vi "readInXml.vi"(8 "error in (no error)":errorcluster, 10 "NativeXML out":refnum<class "NativeXML.lvclass">, 11 "deviceDataBase in":refnum<class "deviceDataBase.lvclass">) -> (0 "error out":errorcluster, 3 "deviceDataBase out":refnum<class "deviceDataBase.lvclass">)   [LabVIEW 2009, in "Tools.lvlib" / "DatabaseHelpers.lvlib" / "deviceDataBase.lvclass"]
uses:
  deviceDataBase.lvclass
  NativeXML/NativeXML.lvclass
  deviceDataBase.lvclass/deviceDataBase.ctl
  Database Objects/DeviceArray/DeviceArray.lvclass
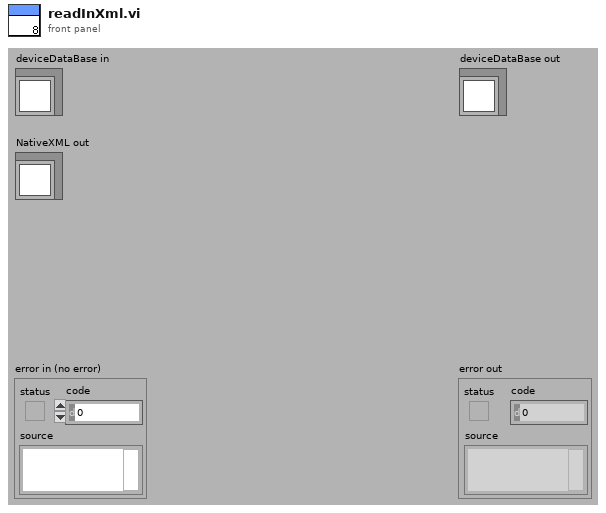
[diagram p1: front panel]
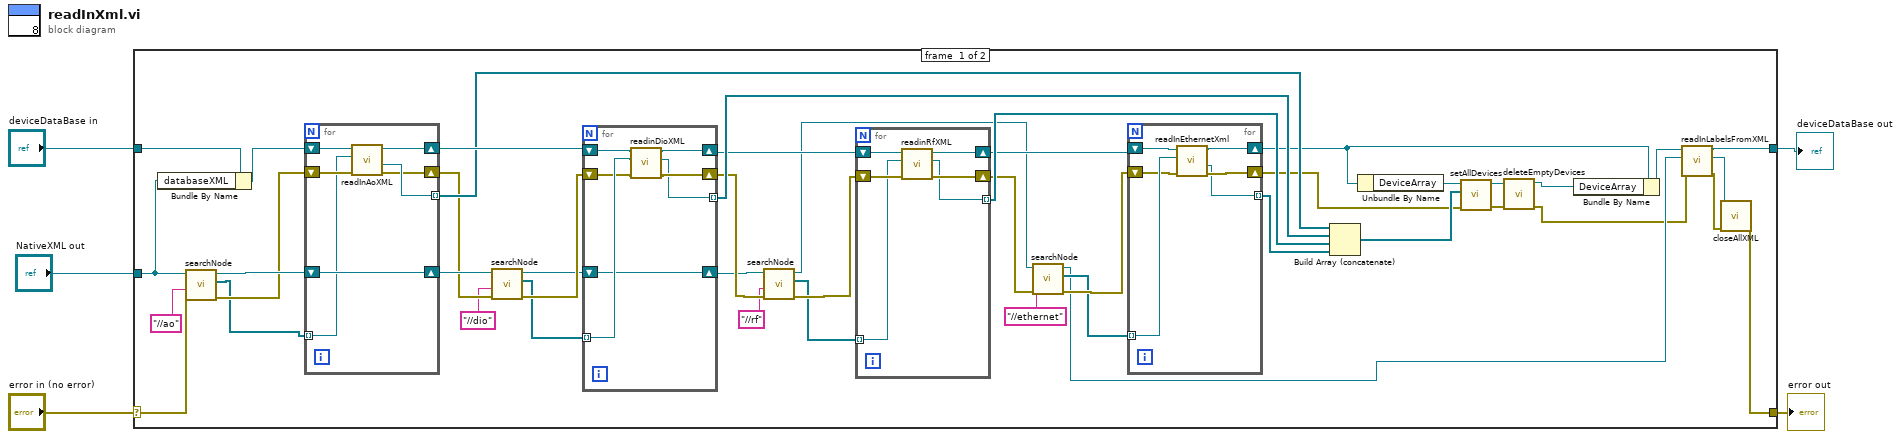
[diagram p0: block diagram]
diagram:
  n1 = case shown="No Error" "error in (no error)" {
    selector: "error in (no error)" -> [w35 w78]
    tunnel: [w7 w78] -> w4
    tunnel: [w6 w77] -> w2
    tunnel: "deviceDataBase in" -> [w50 w77]
    tunnel: "NativeXML out" -> [w32 _]
    frame #0 {
      n2 = Bundle By Name(cluster=w50, "databaseXML"=w32) -> (w49:refnum<class "deviceDataBase.lvclass">)
      n3 = call "searchNode.vi"("error in (no error)"=w35, "searchXPath"="//ao", "NativeXML in"=w32) -> ("error out"=w31:errorcluster, "nodeArray"=w17:refnum<class "NativeXML.lvclass">[], "NativeXML out"=w34:refnum<class "NativeXML.lvclass">)  [unwired: 6 in]
      n4 = for {
        shift-right: [w75] -> w48
        shift-left: w49 -> [w76]
        shift-right: [w71] -> w29
        shift-left: w31 -> [w74]
        tunnel: w17 -> [w70] mode=indexing
        shift-right: [w73] -> w30
        shift-left: w34 -> [w73]
        tunnel: [w72] -> w47 mode=indexing
        n5 = call "readInAoXML.vi"("error in (no error)"=w74, "NativeXML in"=w70, "deviceDataBase in"=w76) -> ("error out"=w71:errorcluster, "device.lvclass out"=w72:refnum<class "device.lvclass">, "deviceDataBase out"=w75:refnum<class "deviceDataBase.lvclass">)  [unwired: 6 in]
      }
      n6 = call "searchNode.vi"("error in (no error)"=w29, "searchXPath"="//dio", "NativeXML in"=w30) -> ("error out"=w27:errorcluster, "nodeArray"=w16:refnum<class "NativeXML.lvclass">[], "NativeXML out"=w26:refnum<class "NativeXML.lvclass">)  [unwired: 6 in]
      n7 = for {
        shift-right: [w68] -> w40
        shift-left: w48 -> [w67]
        shift-right: [w69] -> w24
        shift-left: w27 -> [w65]
        tunnel: w16 -> [w66] mode=indexing
        tunnel: [w64] -> w46 mode=indexing
        shift-right: [w63] -> w23
        shift-left: w26 -> [w63]
        n8 = call "readinDioXML.vi"("error in (no error)"=w65, "channel_configXML"=w66, "deviceDataBase in"=w67) -> ("error out"=w69:errorcluster, "device.lvclass out"=w64:refnum<class "device.lvclass">, "deviceDataBase out"=w68:refnum<class "deviceDataBase.lvclass">)  [unwired: 6 in]
      }
      n9 = call "searchNode.vi"("error in (no error)"=w24, "searchXPath"="//rf", "NativeXML in"=w23) -> ("error out"=w25:errorcluster, "nodeArray"=w15:refnum<class "NativeXML.lvclass">[], "NativeXML out"=w19:refnum<class "NativeXML.lvclass">)  [unwired: 6 in]
      n10 = for {
        shift-right: [w61] -> w38
        shift-left: w40 -> [w62]
        shift-right: [w59] -> w21
        shift-left: w25 -> [w60]
        tunnel: w15 -> [w57] mode=indexing
        tunnel: [w58] -> w39 mode=indexing
        n11 = call "readinRfXML.vi"("error in (no error)"=w60, "xml in"=w57, "deviceDataBase in"=w62) -> ("error out"=w59:errorcluster, "device.lvclass out"=w58:refnum<class "device.lvclass">, "deviceDataBase out"=w61:refnum<class "deviceDataBase.lvclass">)  [unwired: 6 in]
      }
      n12 = call "searchNode.vi"("error in (no error)"=w21, "searchXPath"="//ethernet", "NativeXML in"=w19) -> ("error out"=w22:errorcluster, "nodeArray"=w14:refnum<class "NativeXML.lvclass">[], "NativeXML out"=w11:refnum<class "NativeXML.lvclass">)  [unwired: 6 in]
      n13 = for {
        shift-right: [w55] -> w37
        shift-left: w38 -> [w56]
        shift-right: [w54] -> w13
        shift-left: w22 -> [w51]
        tunnel: w14 -> [w52] mode=indexing
        tunnel: [w53] -> w36 mode=indexing
        n14 = call "readInEthernetXml.vi"("error in (no error)"=w51, "xml in"=w52, "deviceDataBase in"=w56) -> ("error out"=w54:errorcluster, "device.lvclass out"=w53:refnum<class "device.lvclass">, "deviceDataBase out"=w55:refnum<class "deviceDataBase.lvclass">)  [unwired: 6 in]
      }
      n15 = Build Array (concatenate)(w47, w46, w39, w36) -> (w44:refnum<class "device.lvclass">[])
      n16 = Unbundle By Name(w37) -> ("DeviceArray"=w45:refnum<class "DeviceArray.lvclass">)
      n17 = call "setAllDevices.vi"("error in (no error)"=w13, "deviceArray"=w44, "DeviceArray.lvclass in"=w45) -> ("error out"=w43:errorcluster, "DeviceArray.lvclass out"=w42:refnum<class "DeviceArray.lvclass">)  [unwired: 7 in]
      n18 = call "deleteEmptyDevices.vi"("error in (no error)"=w43, "DeviceArray in"=w42) -> ("error out"=w8:errorcluster, "DeviceArray out"=w41:refnum<class "DeviceArray.lvclass">)  [unwired: 8 in]
      n19 = Bundle By Name(cluster=w37, "DeviceArray"=w41) -> (w12:refnum<class "deviceDataBase.lvclass">)
      n20 = call "readInLabelsFromXML.vi"("error in (no error)"=w8, "NativeXML"=w11, "deviceDataBase in"=w12) -> ("error out"=w9:errorcluster, "NativeXML out"=w10:refnum<class "NativeXML.lvclass">, "deviceDataBase out"=w6:refnum<class "deviceDataBase.lvclass">)  [unwired: 6 in]
      n21 = call "closeAllXML.vi"("error in (no error)"=w9, "NativeXML in"=w10) -> ("error out"=w7:errorcluster)  [unwired: 9 in]
    }
    frame #1 {
    }
  }
  "error out" <- w4
  "deviceDataBase out" <- w2
